vi "ConvertStatusRegisterToAxisStatus.vi"(0 "Status":T4, 5 "error in":errorcluster) -> (14 "AxisStatus":T1 {"Drive State Machine" items=["Ready to Switch On"=0, "Fault"=1, "Operation Enabled"=2, "Fault Reaction Active"=3, "Quick Stop Active"=6]}, 19 "error out":errorcluster)   [LabVIEW 2020]
uses:
  General command.llb/Status.ctl
  General command.llb/AxisStatus.ctl
  Special command.llb/DriveStateMachine.ctl
  Special command.llb/ModeOfOperation.ctl
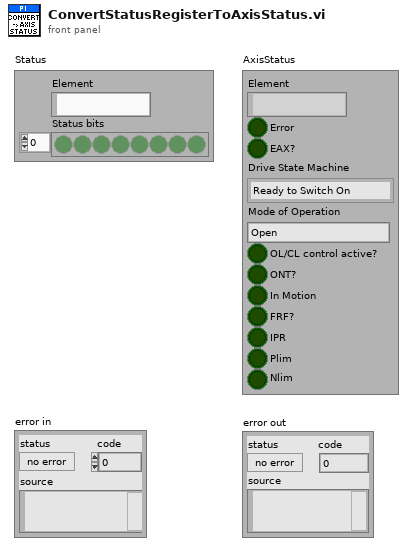
[diagram p1: front panel]
types:
  T1 = typedef "AxisStatus.ctl" = cluster{"Element":string, "Error":bool, "EAX?":bool, "Drive State Machine":T2, "Mode of Operation":T3, "OL/CL control active?":bool, "ONT?":bool, "In Motion":bool, "FRF?":bool, "IPR":bool, "Plim":bool, "Nlim":bool}
  T2 = typedef "DriveStateMachine.ctl" = u16
  T3 = typedef "ModeOfOperation.ctl" = enum16{"Open", "Open-Loop Position", "Closed-Loop Position", "Open-Loop Velocity", "Closed-Loop Velocity", "Open-Loop Force", "Closed-Loop Force", "Step Operation"}
  T4 = typedef "Status.ctl" = cluster{"Element":string, "Status bits":bool[]}
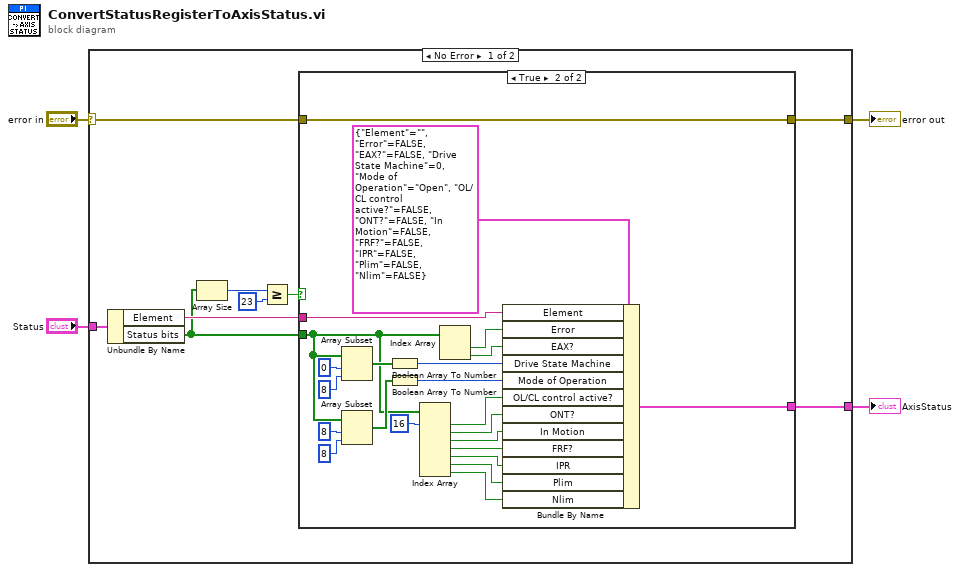
[diagram p0: block diagram]
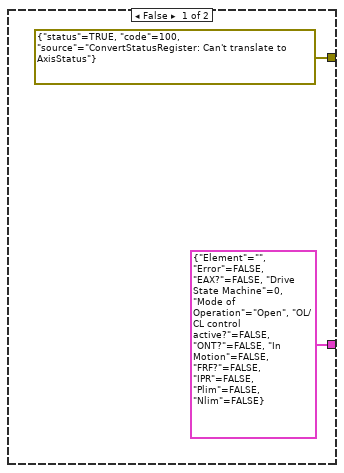
[diagram p2: hidden frame]
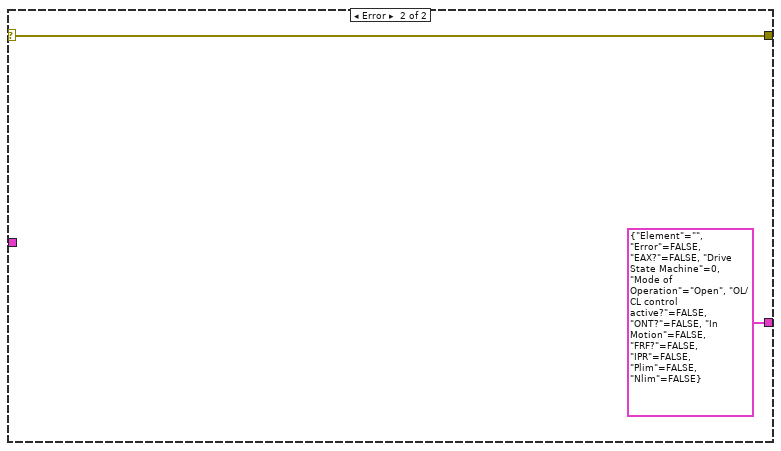
[diagram p3: hidden frame]
diagram:
  n1 = case shown="No Error" "error in" {
    selector: "error in" -> [w8 w40]
    tunnel: [w9 w40] -> w3
    tunnel: "Status" -> [w13 _]
    tunnel: [w5 T1 {"Element"="", "Error"=FALSE, "EAX?"=FALSE, "Drive State Machine"=0, "Mode of Operation"=enum."Open", "OL/CL control active?"=FALSE, "ONT?"=FALSE, "In Motion"=FALSE, "FRF?"=FALSE, "IPR"=FALSE, "Plim"=FALSE, "Nlim"=FALSE} ("AxisStatus")] -> w1
    frame No Error {
      n2 = Unbundle By Name(w13) -> ("Element"=w7:string, "Status bits"=w6:bool[])
      n3 = Array Size(array=w6) -> (size(s)=w10:i32)
      n4 = Greater Or Equal?(x=w10, y=23) -> (x >= y?=w11:bool)
      n5 = case shown="True" w11 {
        tunnel: [errorcluster {"status"=TRUE, "code"=100, "source"="ConvertStatusRegister: Can't translate to AxisStatus"} ("error out") w38] -> w9
        tunnel: w8 -> [_ w38]
        tunnel: w7 -> [_ w20]
        tunnel: w6 -> [_ w19]
        tunnel: [T1 {"Element"="", "Error"=FALSE, "EAX?"=FALSE, "Drive State Machine"=0, "Mode of Operation"=enum."Open", "OL/CL control active?"=FALSE, "ONT?"=FALSE, "In Motion"=FALSE, "FRF?"=FALSE, "IPR"=FALSE, "Plim"=FALSE, "Nlim"=FALSE} ("AxisStatus") w16] -> w5
        frame False {
        }
        frame True {
          n6 = Array Subset(array=w19, index=0, length=8) -> (w29:bool[])
          n7 = Array Subset(array=w19, index=8, length=8) -> (w25:bool[])
          n8 = Boolean Array To Number(Boolean array=w29) -> (number=w22:u32)
          n9 = Boolean Array To Number(Boolean array=w25) -> (number=w26:u32)
          n10 = Index Array(array=w19, index #1=16 ("index")) -> (element #1=w31:bool, element #2=w32:bool, element #3=w33:bool, element #4=w34:bool, element #5=w35:bool, element #6=w36:bool, element #7=w37:bool)  [unwired: 6 in]
          n11 = Index Array(array=w19) -> (element #1=w18:bool, element #2=w17:bool)  [unwired: 2 in]
          n12 = Bundle By Name(cluster=T1 {"Element"="", "Error"=FALSE, "EAX?"=FALSE, "Drive State Machine"=0, "Mode of Operation"=enum."Open", "OL/CL control active?"=FALSE, "ONT?"=FALSE, "In Motion"=FALSE, "FRF?"=FALSE, "IPR"=FALSE, "Plim"=FALSE, "Nlim"=FALSE} ("AxisStatus"), "Element"=w20, "Error"=w18, "EAX?"=w17, "Drive State Machine"=w22, "Mode of Operation"=w26, "OL/CL control active?"=w31, "ONT?"=w32, "In Motion"=w33, "FRF?"=w34, "IPR"=w35, "Plim"=w36, "Nlim"=w37) -> (w16:T1)
        }
      }
    }
    frame Error {
    }
  }
  "error out" <- w3
  "AxisStatus" <- w1
